vi "onGetDefaultPlatanoAppDataFolder.vi"(8 "error in":errorcluster, 11 "Platano in":refnum<class "Platano.lvclass">) -> (0 "error out":errorcluster, 3 "Platano AppData":path)   [LabVIEW 2021, in "Bananas.lvlib" / "Platano.lvclass"]
uses:
  Platano.lvclass
  <vilib>/Utility/sysdir.llb/System Directory Type.ctl
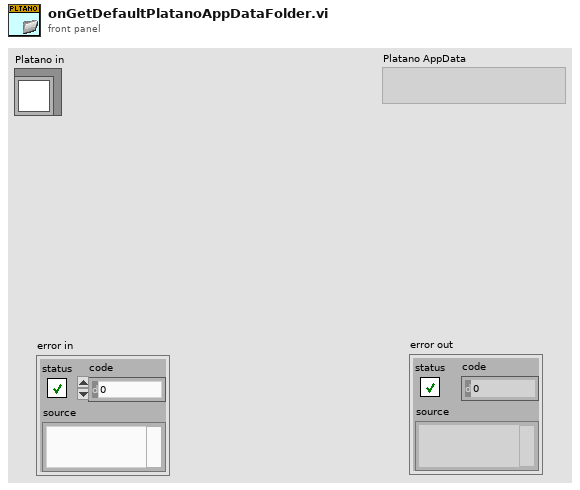
[diagram p1: front panel]
types:
  T1 = typedef "System Directory Type.ctl" = i32
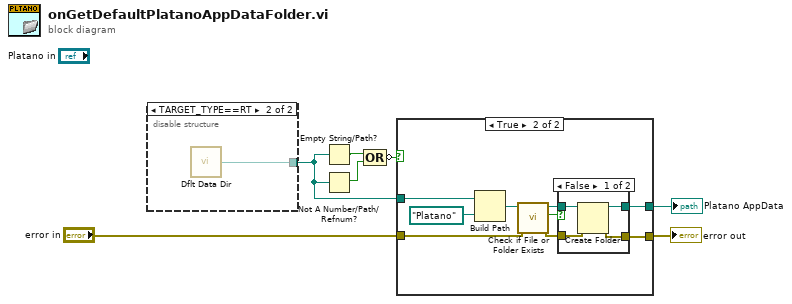
[diagram p0: block diagram]
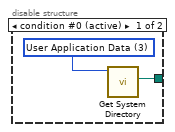
[diagram p2: hidden frame]
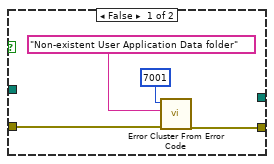
[diagram p3: hidden frame]
diagram:
  n1 = disable-structure shown="TARGET_TYPE==RT" {
    disable-tunnel: [w9 w10] -> w3
    frame condition #0 (active) {
      w8 = T1 3 items=["User Home"=0, "User Desktop"=1, "User Documents"=2, "User Application Data"=3, "User Preferences"=4, "User Temporary"=5, "Public Documents"=6, "Public Application Data"=7, "Public Preferences"=8, "Public Cache"=13, "System Core Libraries"=9, "System Installed Libraries"=10, "Application Files"=11, "Boot Volume Root"=12] ("system directory type")
      n2 = call <vilib>:"Get System Directory.vi"("system directory type"=w8) -> ("system directory"=w9:path)  [unwired: 10 in]
    }
    frame condition #1 {
      n3 = call <vilib>:"Dflt Data Dir.vi"() -> ("App:Default Data Directory"=w10:path)
    }
  }
  n4 = Empty String/Path?(string/path=w3) -> (empty?=w4:bool)
  n5 = Not A Number/Path/Refnum?(number/path/refnum=w3) -> (NaN/Path/Refnum?=w5:bool)
  n6 = Compound Arithmetic op=OR(w4, w5) -> (invert w2:bool)
  n7 = case shown="True" w2 {
    tunnel: w3 -> [_ w22]
    tunnel: [_ w17] -> w6
    tunnel: [w14 w16] -> w7
    tunnel: "error in" -> [w11 w15]
    frame False {
      n8 = call <vilib>:"Error Cluster From Error Code.vi"("error in (no error)"=w11, "error message (\"\")"="Non-existent User Application Data folder" ("error message (\"\")"), "error code (0)"=7001) -> ("error out"=w14:errorcluster)  [unwired: 6 in]
    }
    frame True {
      n9 = Build Path(base path=w22, name or relative path=path "Platano") -> (appended path=w21:path)
      n10 = call <vilib>:"Check if File or Folder Exists.vi"("error in (no error)"=w15, "path"=w21) -> ("error out"=w19:errorcluster, "file or folder exists?"=w18:bool, "dup path"=w20:path)  [unwired: 7 in]
      n11 = case shown="False" w18 {
        tunnel: [w27 w29] -> w17
        tunnel: w20 -> [w26 w29]
        tunnel: w19 -> [w25 w28]
        tunnel: [w24 w28] -> w16
        frame False {
          n12 = Create Folder(path (use dialog)=w26, error in=w25) -> (created path=w27:path, error out=w24:errorcluster)  [unwired: 1 in, 1 out]
        }
        frame True {
        }
      }
    }
  }
  "error out" <- w7
  "Platano AppData" <- w6
